vi "Write TX.vi"(8 "error in (no error)":errorcluster, 10 "TX":string, 11 "PID in":refnum<class "PID.lvclass">) -> (0 "error out":errorcluster, 3 "PID out":refnum<class "PID.lvclass">)   [LabVIEW 2011, in "PID.lvclass"]
uses:
  PID.lvclass
  PID.lvclass/PID.ctl
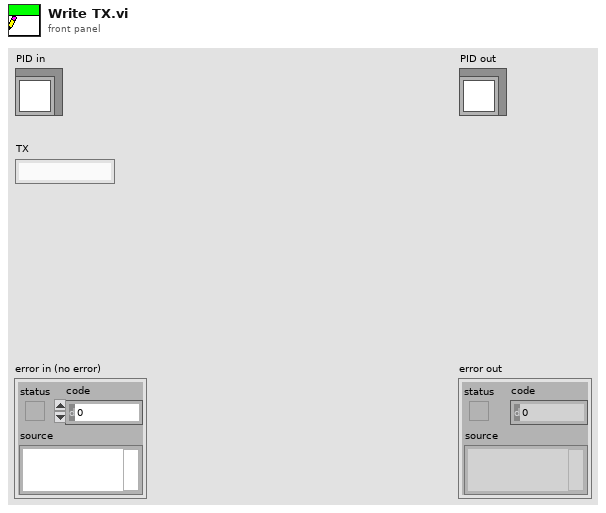
[diagram p1: front panel]
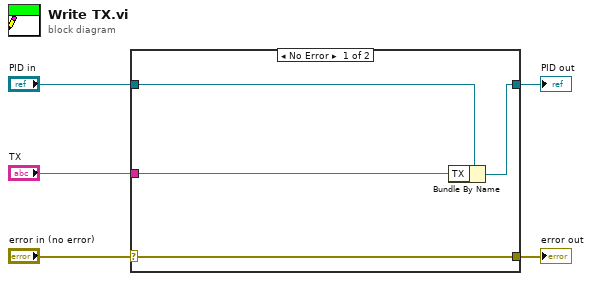
[diagram p0: block diagram]
diagram:
  n1 = case shown="No Error" "error in (no error)" {
    selector: "error in (no error)" -> [w9 w10]
    tunnel: [w9 w10] -> w4
    tunnel: [w7 w11] -> w2
    tunnel: "PID in" -> [w8 w11]
    tunnel: "TX" -> [w6 _]
    frame No Error {
      n2 = Bundle By Name(cluster=w8, "TX"=w6) -> (w7:refnum<class "PID.lvclass">)
    }
    frame Error {
    }
  }
  "error out" <- w4
  "PID out" <- w2
